vi "Freq_Counter.vi"(6 "Maximum Time (10000 ms)":u32=10000, 7 "Count":i32=10, 8 "error in (no error)":errorcluster, 10 "Measurement (0:Frequency)":i32(ring) items=["Frequency", "Frequency Ratio", "Period", "Totalize", "Phase", "Edge Rise Time", "Edge Fall Time", "Positive Pulse Width", "Negative Pulse Width", "Duty Cycle", "Time Interval", "Volt Maximum", "Volt Minimum"], 11 "Counter VISA":refnum<visa-resource-name>) -> (0 "error out":errorcluster, 3 "mean":dbl format="%0.5p")   [LabVIEW 2019]
uses:
  <userlib>/_TI-LA/Instr Drivers/Counter/5313X Series/Driver/Base/Agilent 5313X Series.lvlib
  <vilib>/Analysis/NI_AALBase.lvlib
panel:
  out "standard deviation":dbl format="%0.2f"
  out "Array":dbl[](array[numeric])
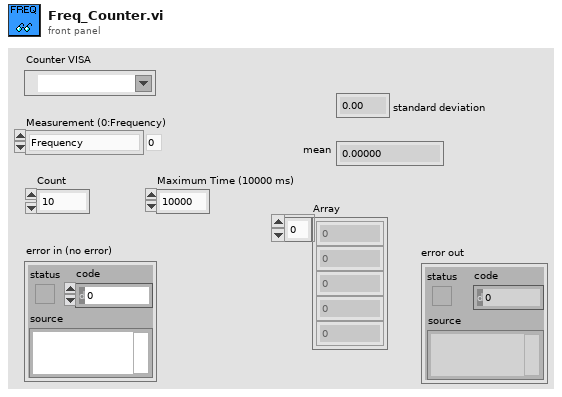
[diagram p1: front panel]
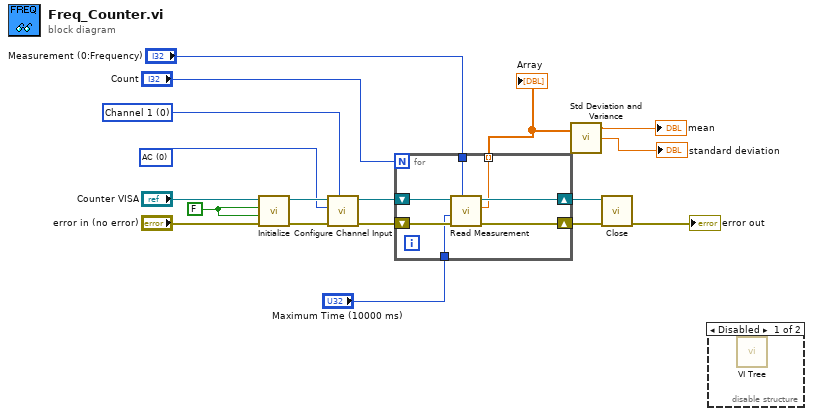
[diagram p0: block diagram]
diagram:
  w7 = FALSE ("ID Query (True)")
  w10 = 0 items=["Channel 1", "Channel 2"] ("Channel (0:Channel 1)")
  w11 = 0 items=["AC", "DC"] ("Coupling (0:AC)")
  n1 = call <userlib>:"Initialize.vi"("error in (no error)"="error in (no error)", "Reset (True)"=w7, "ID Query (True)"=w7, "VISA resource name"="Counter VISA") -> ("error out"=w17:errorcluster, "VISA resource name out"=w18:refnum<visa-resource-name>)  [unwired: 6 in]
  n2 = call <userlib>:"Configure Channel Input.vi"("Channel (0:Channel 1)"=w10, "error in (no error)"=w17, "Coupling (0:AC)"=w11, "VISA resource name"=w18) -> ("error out"=w16:errorcluster, "VISA resource name out"=w15:refnum<visa-resource-name>)  [unwired: 6 in]
  n3 = for {
    N: "Count" -> [_]
    shift-right: [w22] -> w13
    shift-left: w16 -> [w25]
    shift-right: [w23] -> w14
    shift-left: w15 -> [w24]
    tunnel: [w21] -> w3 mode=indexing
    tunnel: "Measurement (0:Frequency)" -> [w20]
    tunnel: "Maximum Time (10000 ms)" -> [w19]
    n4 = call <userlib>:"Read Measurement.vi"("Measurement (0:Frequency)"=w20, "error in (no error)"=w25, "Maximum Time (10000 ms)"=w19, "VISA resource name"=w24) -> ("error out"=w22:errorcluster, "Result"=w21:dbl, "VISA resource name out"=w23:refnum<visa-resource-name>)  [unwired: 5 in]
  }
  "Array" <- w3
  n5 = call <vilib>:"Std Deviation and Variance.vi"("X"=w3) -> ("mean"=→"mean":dbl, "standard deviation"=→"standard deviation":dbl)  [unwired: 1 in, 1 out]
  n6 = call <userlib>:"Close.vi"("error in (no error)"=w13, "VISA resource name"=w14) -> ("error out"=→"error out":errorcluster)  [unwired: 9 in]
  n7 = disable-structure shown="Disabled" {
    frame Disabled {
      n8 = call <userlib>:"VI Tree.vi"() -> ()  [unwired: 12 in]
    }
    frame Enabled {
    }
  }
